vi "WFAppend2.vi"   [LabVIEW 2013]
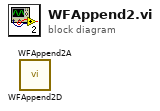
[diagram p0: block diagram]
diagram:
  n1 = call "WFAppend2D.vi"() -> ()  [unwired: 6 in, 2 out]
  n2 = call "WFAppend2A.vi"() -> ()  [unwired: 6 in, 2 out]
